vi "Handle Message.vi"(7 "priority":T1, 8 "error in (no error)":errorcluster, 10 "Message":refnum<class "Message.lvclass">, 11 "Pub Sub Event Channel in":refnum<class "Pub Sub Event Channel.lvclass">) -> (0 "error out":errorcluster)   [LabVIEW 2020, in "Actor Pub Sub Channels.lvlib" / "Pub Sub Event Channel.lvclass"]
uses:
  Pub Sub Event Channel.lvclass
  <vilib>/ActorFramework/Message Dequeuer/Dequeue Priority.ctl
  <vilib>/ActorFramework/Message/Message.lvclass
  Pub Sub Event Channel.lvclass/Pub Sub Event Channel.ctl
  Pub Sub Message Channel/Pub Sub Message Channel.lvclass
  <vilib>/ActorFramework/Message Dequeuer/Message Dequeuer.lvclass
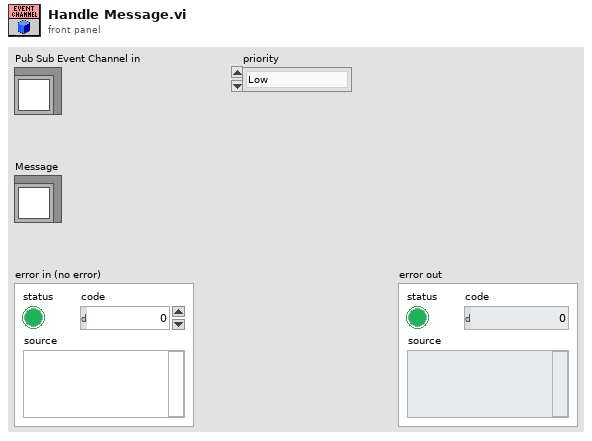
[diagram p1: front panel]
types:
  T1 = typedef "Actor Framework.lvlib/Message Dequeuer.lvclass/Dequeue Priority.ctl" = enum16{"Low", "Normal", "High", "Critical"}
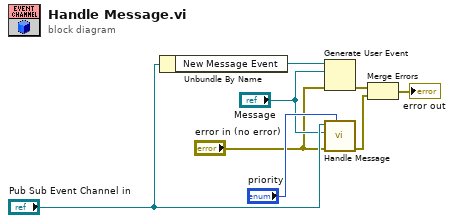
[diagram p0: block diagram]
diagram:
  n1 = Unbundle By Name("Pub Sub Event Channel in") -> ("New Message Event"=w5:refnum<user-event>)
  n2 = Generate User Event(user event=w5, event data cluster="Message", error in="error in (no error)") -> (error out=w1:errorcluster)  [unwired: 1 in, 1 out]
  n3 = call-parent "Handle Message.vi"("priority"="priority", "error in (no error)"="error in (no error)", "Message"="Message", "Pub Sub Message Channel in"="Pub Sub Event Channel in") -> ("error out"=w8:errorcluster)  [unwired: 7 in]
  n4 = Merge Errors(w1, w8) -> (→"error out":errorcluster)
